vi "AddLabel__slk_mt.vi"(8 "error in (no error)":errorcluster, 10 "VI Path":string, 11 "Application Reference":refnum<vi>) -> (0 "error out":errorcluster)   [LabVIEW 2010, in "Lazyboots Menu Tool.lvlib"]
doc: "This VI is the core of <b>Add Label</b> function, and will be called by corresponding menu launcher."
uses:
  Library/Lazyboots Menu Tool.lvlib
  <vilib>/Utility/error.llb/DialogType.ctl
  Private/AddLabel/Class/View/View__slk_mt.lvclass
  Private/AddLabel/Class/Wire/Wire__slk_mt.lvclass
  Private/AddLabel/Class/Label/Label__slk_mt.lvclass
  Private/AddLabel/Class/Segment/Segment__slk_mt.lvclass
panel:
  in  "Ignore Unbefitting":bool
  in  "All Segments":bool
  in  "Segment":u16(ring) items=["Segment 0", "Segment 1", "Segment 2"]
  in  "BG Color":u32(colorbox)=16777215
  in  "Text Color":u32(colorbox)
  in  "Prefix/Postfix":string(combo)=">"
  in  "Label Content":string
  in  "Cancel":bool
  in  "OK":bool
  out "Wire Display":picture
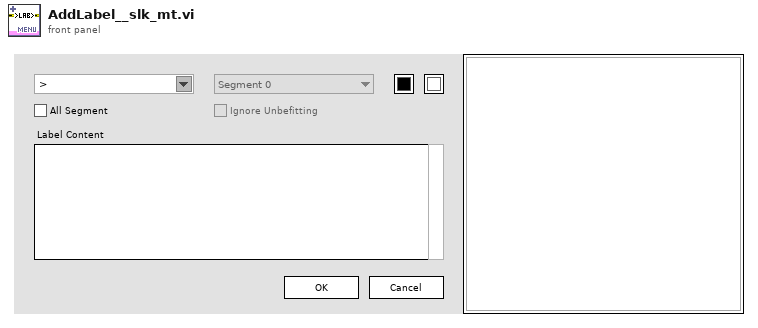
[diagram p1: front panel]
types:
  T1 = enum32{"Invalid", "Standard", "Closed", "Hidden", "Minimized", "Maximized"}
  T2 = cluster{"Width":u16, "Style":enum32{"Solid", "Dash", "Dot", "DashDot", "DashDotDot"}}
  T3 = enum8{"Enabled", "Disabled", "Disabled and Grayed Out"}
  T4 = typedef "DialogType.ctl" = u16
  T5 = typedef "LVRectTypeDef.ctl" = cluster{"Left":i16, "Top":i16, "Right":i16, "Bottom":i16}
  T6 = typedef "LVPoint32TypeDef.ctl" = cluster{"Horizontal":i32, "Vertical":i32}
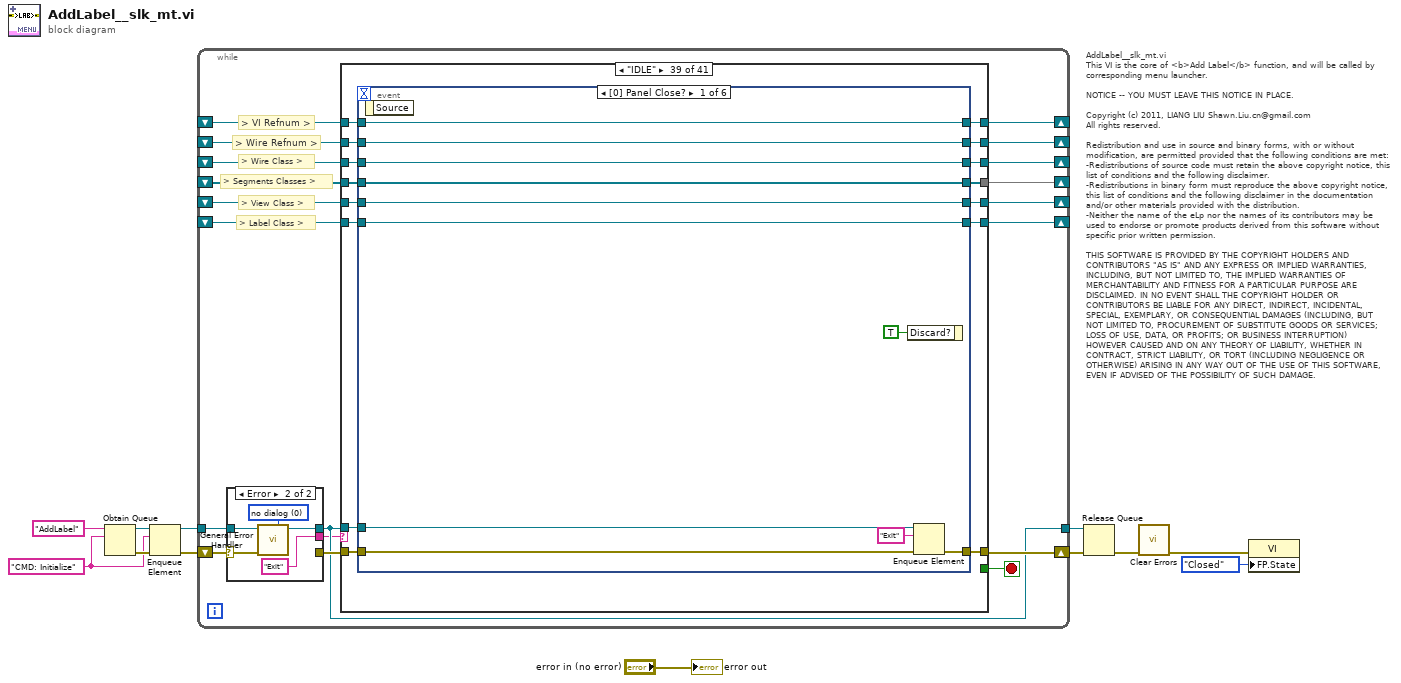
[diagram p0: block diagram]
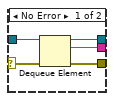
[diagram p2: hidden frame]
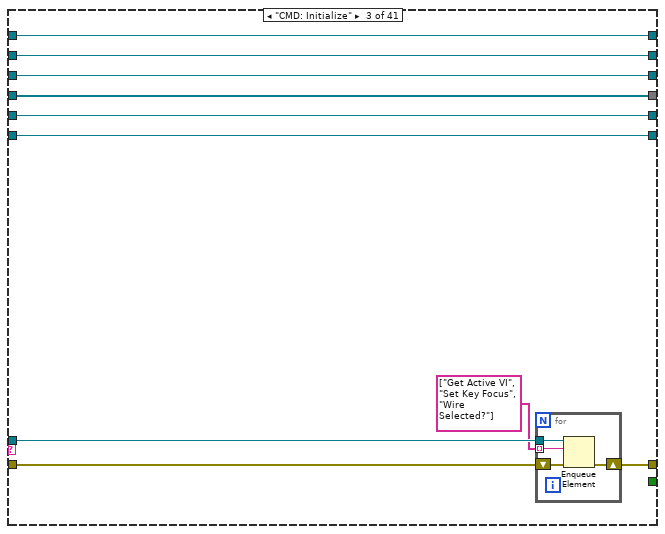
[diagram p5: hidden frame]
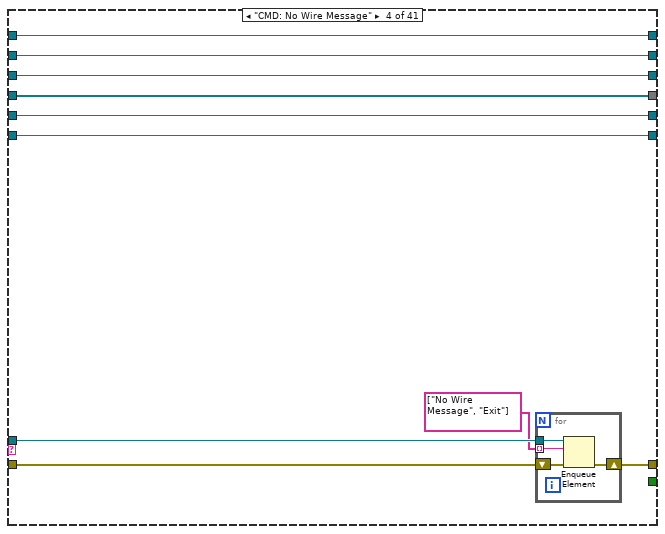
[diagram p6: hidden frame]
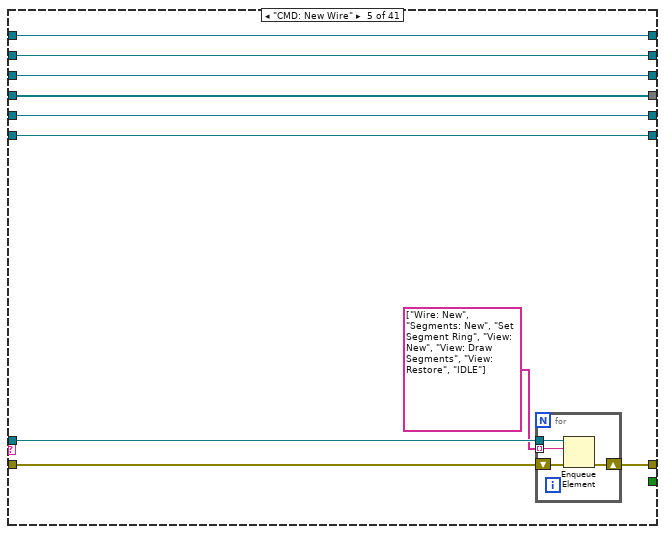
[diagram p7: hidden frame]
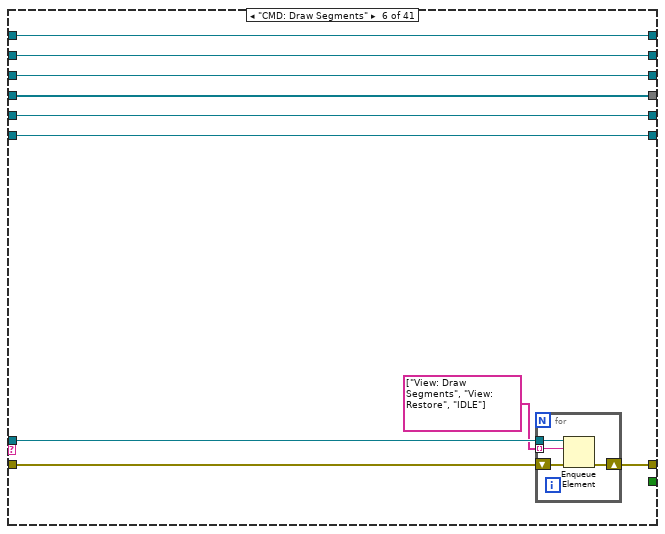
[diagram p8: hidden frame]
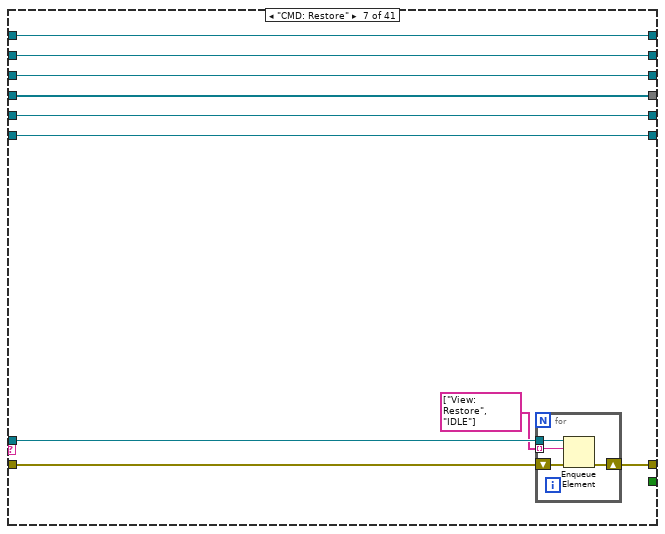
[diagram p9: hidden frame]
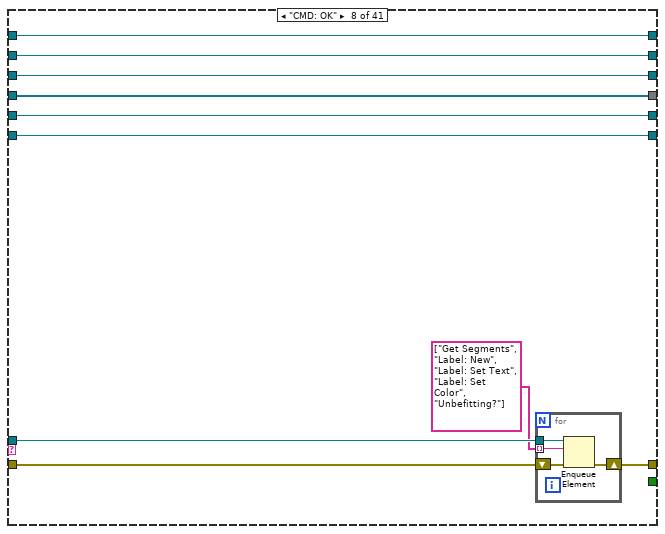
[diagram p10: hidden frame]
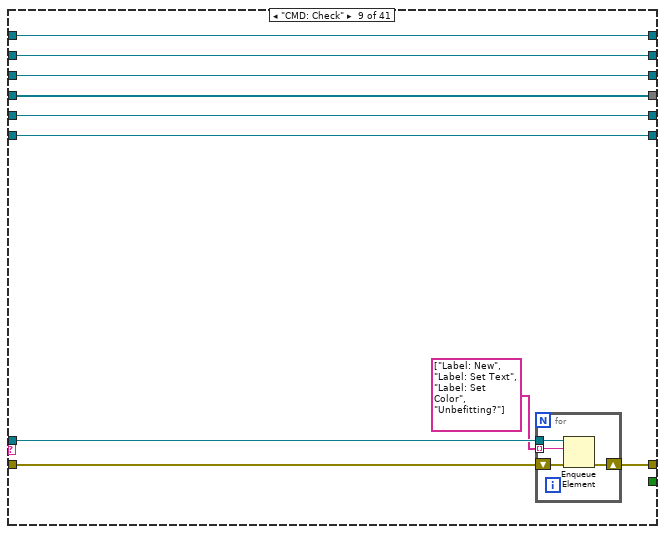
[diagram p11: hidden frame]
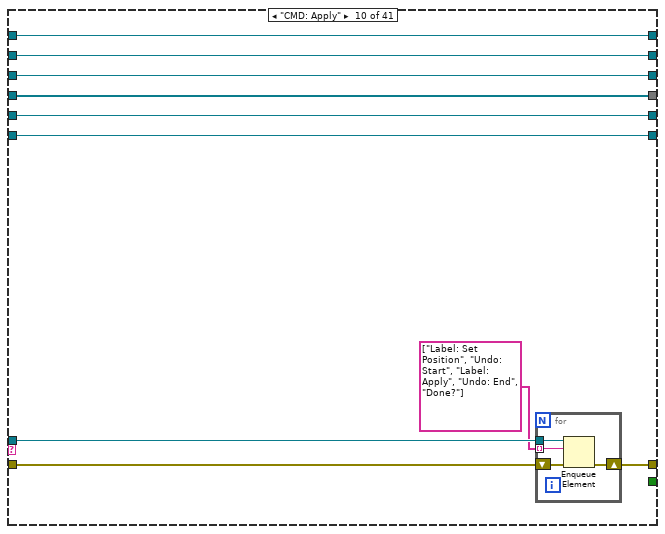
[diagram p12: hidden frame]
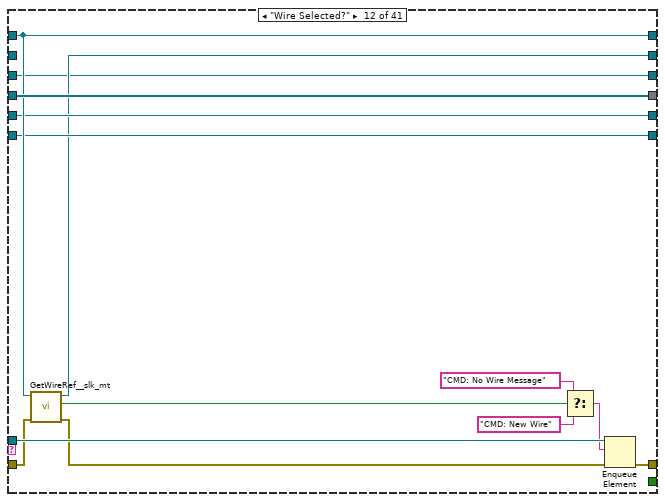
[diagram p14: hidden frame]
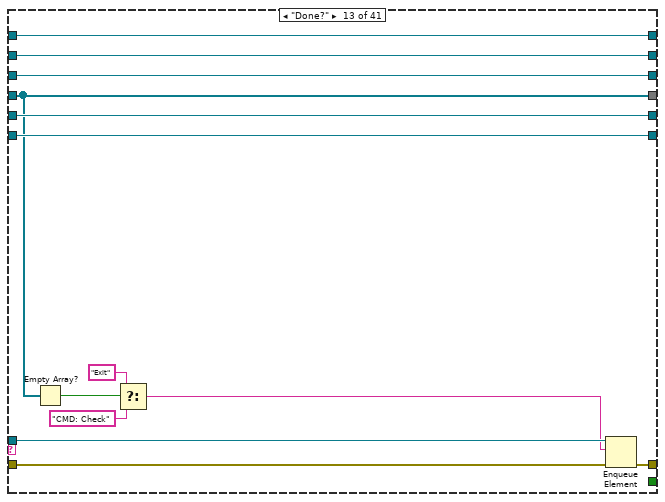
[diagram p15: hidden frame]
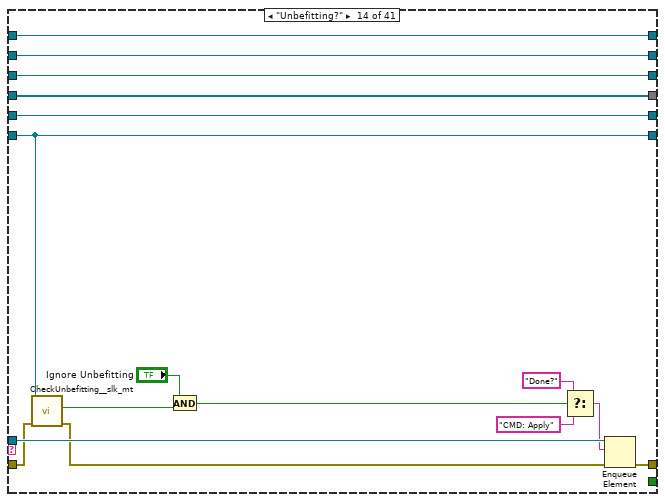
[diagram p16: hidden frame]
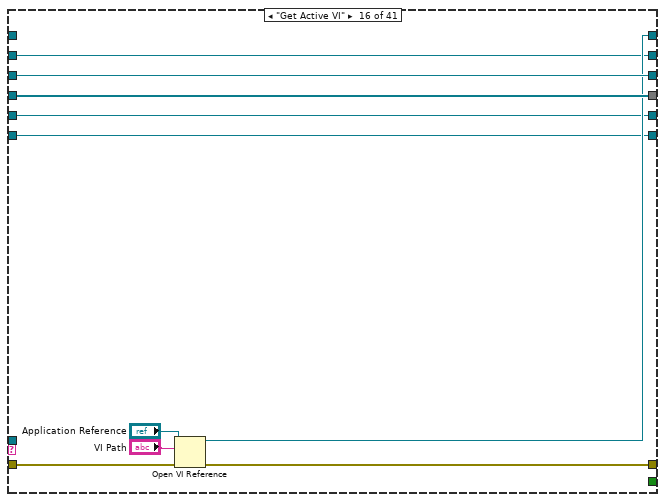
[diagram p18: hidden frame]
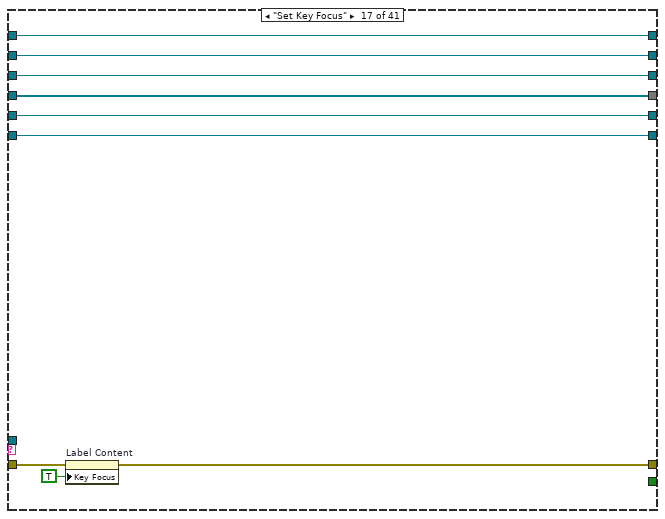
[diagram p19: hidden frame]
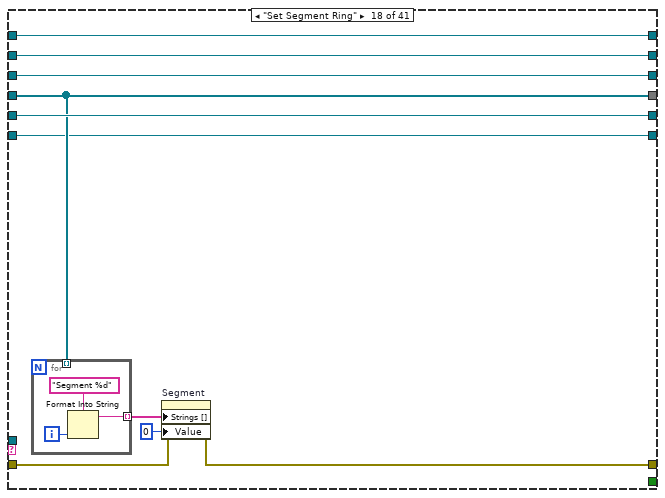
[diagram p20: hidden frame]
diagram:
  w5 = "CMD: Initialize" ("name (unnamed)")
  # "AddLabel__slk_mt.vi\nThis VI is the core of <b>Add Label</b> function, and will be called by corresponding menu launcher.\n\nNOTICE -- YOU MUST LEAVE THIS NOTICE IN PLACE.\n\nCopyright (c) 2011, LIANG LIU Shawn.Liu.cn@gmail.com\nAll rights reserved.\n\nRedistribution and use in source and binary forms, with or without modification, are permitted provided that the following conditions are met:\n-Redistributions of source code must retain the above copyright notice, this list of conditions and the following disclaimer.\n-Redistributions in binary form must reproduce the above copyright notice, this list of conditions and the following disclaimer in the documentation and/or other materials provided with the distribution.\n-Neither the name of the eLp nor the names of its contributors may be used to endorse or promote products derived from this software without specific prior written permission.\n\nTHIS SOFTWARE IS PROVIDED BY THE COPYRIGHT HOLDERS AND CONTRIBUTORS \"AS IS\" AND ANY EXPRESS OR IMPLIED WARRANTIES, INCLUDING, BUT NOT LIMITED TO, THE IMPLIED WARRANTIES OF MERCHANTABILITY AND FITNESS FOR A PARTICULAR PURPOSE ARE DISCLAIMED. IN NO EVENT SHALL THE COPYRIGHT HOLDER OR CONTRIBUTORS BE LIABLE FOR ANY DIRECT, INDIRECT, INCIDENTAL, SPECIAL, EXEMPLARY, OR CONSEQUENTIAL DAMAGES (INCLUDING, BUT NOT LIMITED TO, PROCUREMENT OF SUBSTITUTE GOODS OR SERVICES; LOSS OF USE, DATA, OR PROFITS; OR BUSINESS INTERRUPTION) HOWEVER CAUSED AND ON ANY THEORY OF LIABILITY, WHETHER IN CONTRACT, STRICT LIABILITY, OR TORT (INCLUDING NEGLIGENCE OR OTHERWISE) ARISING IN ANY WAY OUT OF THE USE OF THIS SOFTWARE, EVEN IF ADVISED OF THE POSSIBILITY OF SUCH DAMAGE."
  n1 = Obtain Queue(name (unnamed)="AddLabel", element data type=w5) -> (queue out=w9:refnum<queue>, error out=w10:errorcluster)  [unwired: 3 in, 1 out]
  n2 = Enqueue Element(queue=w9, element=w5, error in (no error)=w10) -> (queue out=w7:refnum<queue>, error out=w6:errorcluster)  [unwired: 2 out]
  n3 = while {
    tunnel: w7 -> [w30]
    shift-right: [w28] -> w12
    shift-left: w6 -> [w31]
    shift-right: [w26] -> _
    shift-left: _ -> [w27]
    shift-right: [w22] -> _
    shift-left: _ -> [w25]
    shift-right: [w23] -> _
    shift-left: _ -> [w24]
    tunnel: [w21] -> w11
    shift-right: [w17] -> _
    shift-left: _ -> [w18]
    shift-right: [w15] -> _
    shift-left: _ -> [w16]
    shift-right: [w13] -> _
    shift-left: _ -> [w14]
    stop <- w20 stop-if-true
    # "> Label Class >"
    # "> View Class >"
    # "> Segments Classes >"
    # "> Wire Class >"
    # "> Wire Refnum >"
    # "> VI Refnum >"
    n4 = case shown="Error" w31 {
      selector: w31 -> [w35 w40]
      tunnel: w30 -> [w36 w39]
      tunnel: [w34 "Exit" ("name (unnamed)")] -> w19
      tunnel: [w33 _] -> w29
      tunnel: [w32 w39] -> w21
      frame No Error {
        n5 = Dequeue Element(queue=w36, error in (no error)=w35) -> (queue out=w32:refnum<queue>, element=w34:string, error out=w33:errorcluster)  [unwired: 2 out]
      }
      frame Error {
        w37 = T4 0 items=["no dialog", "OK message", "continue or stop message", "OK message + warnings", "continue/stop + warnings"] ("type of dialog (OK msg:1)")
        n6 = call <vilib>:"General Error Handler.vi"("type of dialog (OK msg:1)"=w37, "error in (no error)"=w40) -> ()  [unwired: 14 out]
      }
    }
    n7 = case shown="\"IDLE\"" w19 {
      tunnel: w29 -> [w47 w54 w64 w78 w92 w106 w120 w134 w148 w162 w173 w183 w194 w205 w223 w228 w237 w245 w258 w272 w286 w293 w301 w307 w316 w320 w342 w361 w372 w382 w392 w401 w413 w424 w437 w440 w449 w461 w475 w558 w563]
      tunnel: [w47 w54 w57 w71 w85 w99 w113 w127 w141 w155 w173 w186 w196 w215 w223 w226 w234 w243 w256 w272 w286 w287 w301 w302 w316 w317 w326 w356 w372 w373 w386 w399 w412 w423 w437 w438 w447 w461 w474 w558 w561] -> w28
      tunnel: w21 -> [_ _ w56 w70 w84 w98 w112 w126 w140 w154 _ w185 w195 w214 _ _ _ _ _ _ _ _ _ _ _ _ _ _ _ _ _ _ _ _ _ _ _ _ w476 _ _]
      tunnel: w27 -> [w46 w53 w63 w77 w91 w105 w119 w133 w147 w161 w172 w184 w200 w213 w222 _ w238 w252 w266 w279 w285 w290 w300 w309 w315 w325 w346 w365 w371 w385 w398 w411 w422 w427 w436 w442 w450 w460 w473 w557 w569]
      tunnel: [w46 w53 w63 w77 w91 w105 w119 w133 w147 w161 w172 w184 w200 w213 w222 w231 w238 w252 w266 w279 w285 w290 w300 w309 w315 w325 w346 w365 w371 w385 w398 w411 w422 w427 w436 w442 w450 w460 w472 w557 w569] -> w26
      tunnel: w25 -> [w44 w51 w61 w75 w89 w103 w117 w131 w145 w159 w170 w174 w199 w208 w220 w232 w241 w251 w265 w278 w283 _ w298 w304 w313 w324 w330 w358 w369 w381 w396 w409 w420 w429 w434 w445 w453 w458 w471 w555 w559]
      tunnel: w24 -> [w45 w52 w62 w76 w90 w104 w118 w132 w146 w160 w171 w187 w193 w216 w221 w233 w242 w249 w261 w277 w284 w294 w299 _ w314 w323 w344 w364 w370 w376 w395 w408 w418 w430 w435 w446 w452 w459 w470 w556 w568]
      tunnel: [w45 w52 w62 w76 w90 w104 w118 w132 w146 w160 w171 w187 w193 w216 w221 w233 w242 w249 w260 w277 w284 w294 w299 w308 w314 w323 w344 w364 w370 w375 w395 w408 w418 w430 w435 w446 w452 w459 w469 w556 w568] -> w23
      tunnel: [w44 w51 w61 w75 w89 w103 w117 w131 w145 w159 w170 w174 w199 w208 w220 w232 w241 w251 w265 w278 w283 w289 w298 w304 w313 w324 w330 w358 w369 w381 w396 w409 w420 w429 w434 w445 w453 w458 w468 w555 w559] -> w22
      tunnel: [_ _ _ _ _ _ _ _ _ _ _ _ _ _ _ _ _ _ _ _ _ _ _ _ _ _ _ _ _ _ _ _ _ _ _ _ _ _ _ _ TRUE] -> w20
      tunnel: w18 -> [w43 w50 w60 w74 w88 w102 w116 w130 w144 w158 w169 w178 w198 w209 w219 w230 w240 w250 w264 w276 w282 w292 w297 w306 w312 _ w345 w363 w368 w384 w397 w410 w421 w428 w433 w444 w454 w457 w467 w554 w565]
      tunnel: [w43 w50 w60 w74 w88 w102 w116 w130 w144 w158 w169 w178 w198 w209 w219 w230 w240 w250 w264 w276 w282 w292 w297 w306 w312 w321 w345 w363 w368 w384 w397 w410 w421 w428 w433 w444 w454 w457 w466 w554 w565] -> w17
      tunnel: w16 -> [w42 w49 w59 w73 w87 w101 w115 w129 w143 w157 w168 w177 w197 w203 w218 w229 w239 w246 w263 w275 w281 w291 w296 w305 w311 w319 w340 w362 w367 _ w394 w403 w414 w425 w432 w443 w451 w456 w465 w553 w566]
      tunnel: [w42 w49 w59 w73 w87 w101 w115 w129 w143 w157 w168 w177 w197 w203 w218 w229 w239 w246 w263 w275 w281 w291 w296 w305 w311 w319 w340 w362 w367 w383 w388 w402 w419 w425 w432 w443 w451 w456 w464 w553 w566] -> w15
      tunnel: w14 -> [w41 w48 w58 w72 w86 w100 w114 w128 w142 w156 w167 _ w188 w202 w217 w227 w235 w244 w257 w273 w280 w288 w295 w303 w310 w318 w328 w357 w366 w374 w387 w400 w417 w426 w431 w439 w448 w455 w463 w552 w560]
      tunnel: [w41 w48 w58 w72 w86 w100 w114 w128 w142 w156 w167 w175 w188 w202 w217 w227 w235 w244 w257 w273 w280 w288 w295 w303 w310 w318 w328 w357 w366 w374 w387 w400 w417 w426 w431 w439 w448 w455 w462 w552 w560] -> w13
      frame Default {
      }
      frame "----Command----" {
      }
      frame "CMD: Initialize" {
        n8 = for {
          tunnel: w56 -> [w66]
          shift-right: [w67] -> w57
          shift-left: w64 -> [w68]
          tunnel: string[] ["Get Active VI", "Set Key Focus", "Wire Selected?"] -> [w65] mode=indexing
          n9 = Enqueue Element(queue=w66, element=w65, error in (no error)=w68) -> (error out=w67:errorcluster)  [unwired: 1 in, 2 out]
        }
      }
      frame "CMD: No Wire Message" {
        n10 = for {
          tunnel: w70 -> [w80]
          shift-right: [w81] -> w71
          shift-left: w78 -> [w82]
          tunnel: string[] ["No Wire Message", "Exit"] -> [w79] mode=indexing
          n11 = Enqueue Element(queue=w80, element=w79, error in (no error)=w82) -> (error out=w81:errorcluster)  [unwired: 1 in, 2 out]
        }
      }
      frame "CMD: New Wire" {
        n12 = for {
          tunnel: w84 -> [w94]
          shift-right: [w95] -> w85
          shift-left: w92 -> [w96]
          tunnel: string[] ["Wire: New", "Segments: New", "Set Segment Ring", "View: New", "View: Draw Segments", "View: Restore", "IDLE"] -> [w93] mode=indexing
          n13 = Enqueue Element(queue=w94, element=w93, error in (no error)=w96) -> (error out=w95:errorcluster)  [unwired: 1 in, 2 out]
        }
      }
      frame "CMD: Draw Segments" {
        n14 = for {
          tunnel: w98 -> [w108]
          shift-right: [w109] -> w99
          shift-left: w106 -> [w110]
          tunnel: string[] ["View: Draw Segments", "View: Restore", "IDLE"] -> [w107] mode=indexing
          n15 = Enqueue Element(queue=w108, element=w107, error in (no error)=w110) -> (error out=w109:errorcluster)  [unwired: 1 in, 2 out]
        }
      }
      frame "CMD: Restore" {
        n16 = for {
          tunnel: w112 -> [w122]
          shift-right: [w123] -> w113
          shift-left: w120 -> [w124]
          tunnel: string[] ["View: Restore", "IDLE"] -> [w121] mode=indexing
          n17 = Enqueue Element(queue=w122, element=w121, error in (no error)=w124) -> (error out=w123:errorcluster)  [unwired: 1 in, 2 out]
        }
      }
      frame "CMD: OK" {
        n18 = for {
          tunnel: w126 -> [w136]
          shift-right: [w137] -> w127
          shift-left: w134 -> [w138]
          tunnel: string[] ["Get Segments", "Label: New", "Label: Set Text", "Label: Set Color", "Unbefitting?"] -> [w135] mode=indexing
          n19 = Enqueue Element(queue=w136, element=w135, error in (no error)=w138) -> (error out=w137:errorcluster)  [unwired: 1 in, 2 out]
        }
      }
      frame "CMD: Check" {
        n20 = for {
          tunnel: w140 -> [w150]
          shift-right: [w151] -> w141
          shift-left: w148 -> [w152]
          tunnel: string[] ["Label: New", "Label: Set Text", "Label: Set Color", "Unbefitting?"] -> [w149] mode=indexing
          n21 = Enqueue Element(queue=w150, element=w149, error in (no error)=w152) -> (error out=w151:errorcluster)  [unwired: 1 in, 2 out]
        }
      }
      frame "CMD: Apply" {
        n22 = for {
          tunnel: w154 -> [w164]
          shift-right: [w165] -> w155
          shift-left: w162 -> [w166]
          tunnel: string[] ["Label: Set Position", "Undo: Start", "Label: Apply", "Undo: End", "Done?"] -> [w163] mode=indexing
          n23 = Enqueue Element(queue=w164, element=w163, error in (no error)=w166) -> (error out=w165:errorcluster)  [unwired: 1 in, 2 out]
        }
      }
      frame "----Query----" {
      }
      frame "Wire Selected?" {
        n24 = call "GetWireRef__slk_mt.vi"("error in (no error)"=w183, "vi refnum in"=w184) -> ("error out"=w176:errorcluster, "not found?"=w179:bool, "wire refnum out"=w175:refnum<vi>)  [unwired: 7 in]
        n25 = Select(t="CMD: No Wire Message" ("element"), s=w179, f="CMD: New Wire" ("element")) -> (s? t:f=w180:string)
        n26 = Enqueue Element(queue=w185, element=w180, error in (no error)=w176) -> (error out=w186:errorcluster)  [unwired: 3 out]
      }
      frame "Done?" {
        n27 = Empty Array?(array=w193) -> (empty?=w192:bool)
        n28 = Select(t="Exit" ("element"), s=w192, f="CMD: Check" ("element")) -> (s? t:f=w189:string)
        n29 = Enqueue Element(queue=w195, element=w189, error in (no error)=w194) -> (error out=w196:errorcluster)  [unwired: 1 in, 2 out]
      }
      frame "Unbefitting?" {
        n30 = call "CheckUnbefitting__slk_mt.vi"("error in (no error)"=w205, "label in"=w203) -> ("error out"=w204:errorcluster, "unbefitting?"=w206:bool)  [unwired: 7 in, 1 out]
        n31 = And(x="Ignore Unbefitting", y=w206) -> (x .and. y?=w201:bool)
        n32 = Select(t="Done?" ("element"), s=w201, f="CMD: Apply" ("element")) -> (s? t:f=w210:string)
        n33 = Enqueue Element(queue=w214, element=w210, error in (no error)=w204) -> (error out=w215:errorcluster)  [unwired: 3 out]
      }
      frame "----Add Label----" {
      }
      frame "Get Active VI" {
        n34 = Open VI Reference(application reference (local)="Application Reference", vi path="VI Path", error in (no error)=w228) -> (vi reference=w231:refnum<vi>, error out=w226:errorcluster)  [unwired: 3 out]
      }
      frame "Set Key Focus" {
        n35 = property on="Label Content" class="Str"(error in=w237, "Key Focus"=TRUE) -> (error out=w234:errorcluster)  [unwired: 1 in, 1 out]
      }
      frame "Set Segment Ring" {
        n36 = for {
          tunnel: w249 -> [_] mode=indexing
          tunnel: [w253] -> w248 mode=indexing
          i -> [w255]
          n37 = Format Into String(format string="Segment %d", w255) -> (resulting string=w253:string)  [unwired: 2 in, 1 out]
        }
        n38 = property on="Segment" class="Ring (strict)"(error in=w245, "Strings []"=w248, "Value"=u16 0) -> (error out=w243:errorcluster)  [unwired: 1 in, 1 out]
      }
      frame "Get Segments" {
        n39 = property on="Segment" class="Ring (strict)"(error in=w258) -> (error out=w256:errorcluster, "Value"=w259:u16)  [unwired: 1 in, 1 out]
        n40 = case shown="False" "All Segments" {
          tunnel: w261 -> [w270 w271]
          tunnel: [w269 w271] -> w260
          tunnel: w259 -> [w268 _]
          frame False {
            n41 = Array Subset(array=w270, index=w268, length=1) -> (w269:refnum<class "Segment__slk_mt.lvclass">[])
          }
          frame True {
          }
        }
      }
      frame "No Wire Message" {
        n42 = One Button Dialog(message="There is no wire in selection list, please select a wire first!") -> ()  [unwired: 2 out]
      }
      frame "----Wire----" {
      }
      frame "Wire: New" {
        n43 = call "New__slk_mt.vi"("error in (no error)"=w293, "wire refnum in"=w288) -> ("error out"=w287:errorcluster, "wire out"=w289:refnum<class "Wire__slk_mt.lvclass">)  [unwired: 8 in]
      }
      frame "----Segment----" {
      }
      frame "Segments: New" {
        n44 = call "GetSegments__slk_mt.vi"("error in (no error)"=w307, "wire in"=w304) -> ("error out"=w302:errorcluster, "segments"=w308:refnum<class "Segment__slk_mt.lvclass">[])  [unwired: 7 in, 1 out]
      }
      frame "----View----" {
      }
      frame "View: New" {
        n45 = control-ref of="Wire Display"() -> (w322:refnum<vi>)
        n46 = call "New__slk_mt.vi"("error in (no error)"=w320, "picture refnum in"=w322) -> ("error out"=w317:errorcluster, "view out"=w321:refnum<class "View__slk_mt.lvclass">)  [unwired: 8 in]
      }
      frame "View: Draw Segments" {
        n47 = call "Delete__slk_mt.vi"("error in (no error)"=w342, "view in"=w345) -> ("error out"=w341:errorcluster, "view out"=w343:refnum<class "View__slk_mt.lvclass">)  [unwired: 8 in]
        n48 = for {
          shift-right: [w355] -> w337
          shift-left: w341 -> [w351]
          tunnel: w343 -> [w354]
          tunnel: w344 -> [w352] mode=indexing
          tunnel: [w353] -> w339
          tunnel: T2 {"Width"=1, "Style"=enum."Dot"} ("pen") -> [w348]
          tunnel: u32 32639 ("color") -> [w347]
          n49 = call "GetJoints__slk_mt.vi"("error in (no error)"=w351, "segment in"=w352) -> ("error out"=w350:errorcluster, "Joints"=w349:cluster{"X":i32, "Y":i32}[])  [unwired: 7 in, 1 out]
          n50 = call "DrawSegment__slk_mt.vi"("color"=w347, "pen"=w348, "error in (no error)"=w350, "joints"=w349, "view in"=w354) -> ("error out"=w355:errorcluster, "view out"=w353:refnum<class "View__slk_mt.lvclass">)  [unwired: 5 in]
        }
        n51 = To Long Integer(number="Segment") -> (32bit integer=w329:i32)
        n52 = Index Array(array=w344, index=w329) -> (element=w338:refnum<class "Segment__slk_mt.lvclass">)
        n53 = call "GetJoints__slk_mt.vi"("error in (no error)"=w337, "segment in"=w338) -> ("error out"=w336:errorcluster, "Joints"=w335:cluster{"X":i32, "Y":i32}[])  [unwired: 7 in, 1 out]
        n54 = call "DrawSegment__slk_mt.vi"("color"=u32 16711680, "pen"=T2 {"Width"=2, "Style"=enum."Solid"}, "error in (no error)"=w336, "joints"=w335, "view in"=w339) -> ("error out"=w326:errorcluster)  [unwired: 5 in, 1 out]
      }
      frame "View: Restore" {
        n55 = call "GetTotalBoundsRectangle__slk_mt.vi"("error in (no error)"=w361, "wire in"=w358) -> ("error out"=w360:errorcluster, "rectangle"=w359:T5)  [unwired: 7 in, 1 out]
        n56 = call "FitToDrawArea__slk_mt.vi"("error in (no error)"=w360, "total bounds"=w359, "view in"=w363) -> ("error out"=w356:errorcluster)  [unwired: 7 in, 1 out]
      }
      frame "----Label----" {
      }
      frame "Label: New" {
        n57 = Delete From Array(array=w376, length=1, index=0) -> (deleted portion=w377:refnum<class "Segment__slk_mt.lvclass">[], array with subset deleted=w375:refnum<class "Segment__slk_mt.lvclass">[])
        n58 = Index Array(array=w377) -> (element=w380:refnum<class "Segment__slk_mt.lvclass">)  [unwired: 1 in]
        n59 = call "New__slk_mt.vi"("error in (no error)"=w382, "segment in"=w380) -> ("error out"=w373:errorcluster, "label out"=w383:refnum<class "Label__slk_mt.lvclass">)  [unwired: 8 in]
      }
      frame "Label: Set Text" {
        n60 = call "SetPrefixPostfix__slk_mt.vi"("error in (no error)"=w392, "prefix/postfix"="Prefix/Postfix", "label in"=w394) -> ("error out"=w391:errorcluster, "label out"=w390:refnum<class "Label__slk_mt.lvclass">)  [unwired: 7 in]
        n61 = call "SetText__slk_mt.vi"("error in (no error)"=w391, "text"="Label Content", "label in"=w390) -> ("error out"=w386:errorcluster, "label out"=w388:refnum<class "Label__slk_mt.lvclass">)  [unwired: 7 in]
      }
      frame "Label: Set Color" {
        n62 = call "SetTextColor__slk_mt.vi"("error in (no error)"=w401, "text color"="Text Color", "label in"=w403) -> ("error out"=w407:errorcluster, "label out"=w406:refnum<class "Label__slk_mt.lvclass">)  [unwired: 7 in]
        n63 = call "SetBGColor__slk_mt.vi"("error in (no error)"=w407, "bg color"="BG Color", "label in"=w406) -> ("error out"=w399:errorcluster, "label out"=w402:refnum<class "Label__slk_mt.lvclass">)  [unwired: 7 in]
      }
      frame "Label: Set Position" {
        n64 = call "SetPosition__slk_mt.vi"("error in (no error)"=w413, "label in"=w414) -> ("error out"=w416:errorcluster, "label out"=w415:refnum<class "Label__slk_mt.lvclass">)  [unwired: 8 in]
        n65 = call "SetVerticalArrangement__slk_mt.vi"("error in (no error)"=w416, "label in"=w415) -> ("error out"=w412:errorcluster, "label out"=w419:refnum<class "Label__slk_mt.lvclass">)  [unwired: 8 in]
      }
      frame "Label: Apply" {
        n66 = call "Apply__slk_mt.vi"("error in (no error)"=w424, "label in"=w425) -> ("error out"=w423:errorcluster)  [unwired: 8 in, 1 out]
      }
      frame "----Undo----" {
      }
      frame "Undo: Start" {
        n67 = invoke class="VI" method="Transaction.Begin Undo"(reference=w442, error in=w440, "Name"="AddLabel__slk_mt") -> (error out=w438:errorcluster)  [unwired: 1 in, 3 out]
      }
      frame "Undo: End" {
        n68 = invoke class="VI" method="Transaction.End Undo"(reference=w450, error in=w449) -> (error out=w447:errorcluster)  [unwired: 1 in, 2 out]
      }
      frame "----Event----" {
      }
      frame "IDLE" {
        n69 = event shown="[0] Panel Close?" {
          selector: _ -> [_ _ _ _ _ _]
          dyn-events: _ -> [_ _ _ _ _ _]
          timeout: _ -> [_ _ _ _ _ _]
          tunnel: w476 -> [w481 w495 w501 w511 w527 w549]
          tunnel: w475 -> [w484 w490 w504 w514 w518 w544]
          tunnel: [w482 w496 w502 w512 w528 w550] -> w474
          tunnel: w473 -> [w487 w497 w507 w517 w532 w551]
          tunnel: [w487 w497 w507 w517 w532 w551] -> w472
          tunnel: w471 -> [w486 w491 w506 w516 w531 w548]
          tunnel: w470 -> [w485 w492 w505 w515 w530 w543]
          tunnel: [w485 w492 w505 w515 w530 w543] -> w469
          tunnel: [w486 w491 w506 w516 w531 w548] -> w468
          tunnel: w467 -> [w483 w493 w503 w513 w529 w542]
          tunnel: [w483 w493 w503 w513 w529 w542] -> w466
          tunnel: w465 -> [w479 w489 w499 w509 w525 w547]
          tunnel: [w479 w489 w499 w509 w525 w547] -> w464
          tunnel: w463 -> [w478 w488 w498 w508 w519 w546]
          tunnel: [w478 w488 w498 w508 w519 w546] -> w462
          event Panel Close? {
            n70 = event-data() -> ()  [unwired: 2 out]
            n71 = event-data("Discard?"=TRUE) -> ()  [unwired: 1 in, 1 out]
            n72 = Enqueue Element(queue=w481, element="Exit", error in (no error)=w484) -> (error out=w482:errorcluster)  [unwired: 1 in, 2 out]
          }
          event Panel Resize {
            n73 = event-data() -> ()  [unwired: 2 out]
            n74 = Enqueue Element(queue=w495, element="CMD: Restore", error in (no error)=w490) -> (error out=w496:errorcluster)  [unwired: 1 in, 2 out]
          }
          event "Cancel": Value Change {
            n75 = event-data() -> ()  [unwired: 2 out]
            n76 = Enqueue Element(queue=w501, element="Exit", error in (no error)=w504) -> (error out=w502:errorcluster)  [unwired: 1 in, 2 out]
          }
          event "OK": Value Change {
            n77 = event-data() -> ()  [unwired: 2 out]
            n78 = Enqueue Element(queue=w511, element="CMD: OK", error in (no error)=w514) -> (error out=w512:errorcluster)  [unwired: 1 in, 2 out]
          }
          event "All Segments": Value Change {
            n79 = event-data() -> ("NewVal"=w522:bool)  [unwired: 1 out]
            n80 = Select(t=T3."Enabled" ("Disabled"), s=w522, f=T3."Disabled and Grayed Out" ("Disabled")) -> (s? t:f=w523:T3)
            n81 = property on="Ignore Unbefitting" class="Bool (strict)"(error in=w518, "DisabledEnum"=w523) -> (error out=w524:errorcluster)  [unwired: 1 in, 1 out]
            n82 = Enqueue Element(queue=w527, element="IDLE", error in (no error)=w524) -> (error out=w528:errorcluster)  [unwired: 1 in, 2 out]
          }
          event "Wire Display": Mouse Down {
            n83 = event-data() -> ("Coords"=w540:T6)  [unwired: 1 out]
            n84 = call "InRanges__slk_mt.vi"("segments in"=w543, "error in (no error)"=w544, "point"=w540, "view in"=w542) -> ("error out"=w541:errorcluster, "range index"=w539:u16, "in ranges?"=w537:bool)  [unwired: 5 in]
            n85 = Select(t=w539, s=w537, f=u16 0) -> (s? t:f=w538:u16)
            n86 = Select(t="CMD: Draw Segments" ("element"), s=w537, f="IDLE" ("element")) -> (s? t:f=w534:string)
            n87 = To Unsigned Word Integer(number=w538) -> (unsigned 16bit integer=w545:u16)
            n88 = property on="Segment" class="Ring (strict)"("Value"=w545) -> ()  [unwired: 2 in, 2 out]
            n89 = Enqueue Element(queue=w549, element=w534, error in (no error)=w541) -> (error out=w550:errorcluster)  [unwired: 1 in, 2 out]
          }
        }
      }
      frame "----Exit----" {
      }
      frame "Exit" {
        n90 = call "Close__slk_mt.vi"("error in (no error)"=w563, "view in"=w565) -> ("error out"=w564:errorcluster)  [unwired: 9 in]
        n91 = call "Close__slk_mt.vi"("error in (no error)"=w564, "wire in"=w559) -> ("error out"=w562:errorcluster)  [unwired: 9 in]
        n92 = call <vilib>:"Clear Errors.vi"("error in (no error)"=w562) -> ("error out"=w561:errorcluster)  [unwired: 6 in]
      }
    }
  }
  n93 = Release Queue(queue=w11, error in (no error)=w12) -> (error out=w3:errorcluster)  [unwired: 3 out]
  n94 = call <vilib>:"Clear Errors.vi"("error in (no error)"=w3) -> ("error out"=w4:errorcluster)  [unwired: 6 out]
  n95 = property class="VI"(error in=w4, "FP.State"=T1."Closed" ("Front Panel Window:State")) -> ()  [unwired: 1 in, 2 out]
  "error out" <- "error in (no error)"
